vi "Binary Post-Uninstall Custom Action.vi"(10 "Variant":variant) -> (0 "error out":errorcluster)   [LabVIEW 2020]
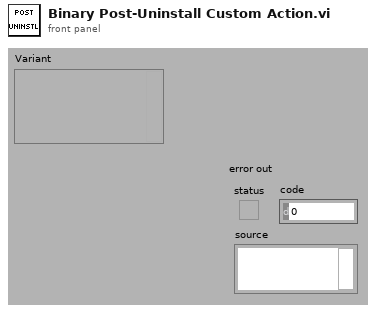
[diagram p1: front panel]
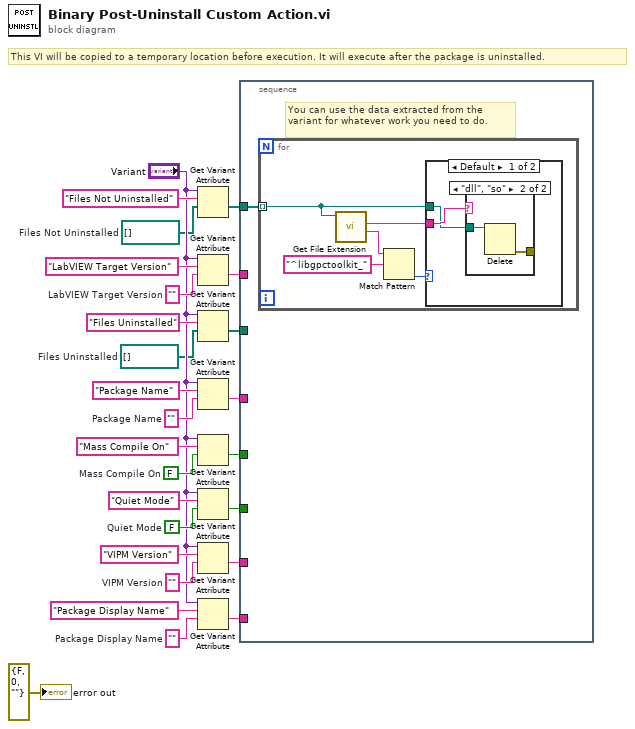
[diagram p0: block diagram]
diagram:
  w1 = path[] []  # Files Not Uninstalled
  w2 = path[] []  # Files Uninstalled
  w8 = FALSE  # Mass Compile On
  w9 = ""  # Package Display Name
  w16 = FALSE  # Quiet Mode
  w19 = ""  # VIPM Version
  w21 = ""  # LabVIEW Target Version
  w23 = ""  # Package Name
  # "This VI will be copied to a temporary location before execution. It will execute after the package is uninstalled."
  n1 = Get Variant Attribute(Variant="Variant", name="Files Not Uninstalled", default value (empty Variant)=w1) -> (value=w6:path[])  [unwired: 1 in, 3 out]
  n2 = Get Variant Attribute(Variant="Variant", name="LabVIEW Target Version", default value (empty Variant)=w21) -> (value=w13:string)  [unwired: 1 in, 3 out]
  n3 = Get Variant Attribute(Variant="Variant", name="Files Uninstalled", default value (empty Variant)=w2) -> (value=w5:path[])  [unwired: 1 in, 3 out]
  n4 = Get Variant Attribute(Variant="Variant", name="Package Name", default value (empty Variant)=w23) -> (value=w14:string)  [unwired: 1 in, 3 out]
  n5 = Get Variant Attribute(Variant="Variant", name="Mass Compile On", default value (empty Variant)=w8) -> (value=w10:bool)  [unwired: 1 in, 3 out]
  n6 = Get Variant Attribute(Variant="Variant", name="Quiet Mode", default value (empty Variant)=w16) -> (value=w11:bool)  [unwired: 1 in, 3 out]
  n7 = Get Variant Attribute(Variant="Variant", name="VIPM Version", default value (empty Variant)=w19) -> (value=w12:string)  [unwired: 1 in, 3 out]
  n8 = Get Variant Attribute(Variant="Variant", name="Package Display Name", default value (empty Variant)=w9) -> (value=w15:string)  [unwired: 1 in, 3 out]
  n9 = stacked-sequence {
    tunnel: w15 -> [_]
    tunnel: w14 -> [_]
    tunnel: w13 -> [_]
    tunnel: w12 -> [_]
    tunnel: w11 -> [_]
    tunnel: w10 -> [_]
    tunnel: w5 -> [_]
    tunnel: w6 -> [w27]
    frame #0 {
      # "You can use the data extracted from the variant for whatever work you need to do."
      n10 = for {
        tunnel: w27 -> [w28] mode=indexing
        n11 = call <vilib>:"Get File Extension.vi"("file"=w28) -> ("filename without extension"=w32:string, "lowercase file extension"=w29:string)  [unwired: 6 in, 3 out]
        n12 = Match Pattern(string=w32, regular expression="^libgpctoolkit_") -> (offset past match=w30:i32)  [unwired: 1 in, 3 out]
        n13 = case shown="Default" w30 {
          tunnel: w29 -> [w34 _]
          tunnel: w28 -> [w33 _]
          frame Default {
            n14 = case shown="\"dll\", \"so\"" w34 {
              tunnel: w33 -> [_ w36]
              tunnel: [_ w35] -> _
              frame "False", Default {
              }
              frame "dll", "so" {
                n15 = Delete(path (use dialog)=w36) -> (error out=w35:errorcluster)  [unwired: 4 in, 2 out]
              }
            }
          }
          frame -1 {
          }
        }
      }
    }
  }
  "error out" <- errorcluster {"status"=FALSE, "code"=0, "source"=""} ("error out")
